vi "RC steering control.vi"(8 "filterd chan 0":dbl, 9 "Control with RC":bool, 10 "Duty Cycle in":dbl(slide) scale=0.0..1.0, 11 "Switch direction in":bool) -> (0 "Switch direction out":bool, 2 "Duty Cycle out":dbl)   [LabVIEW 2016]
doc: "Input\nChannel 0 data\nControl with RC\nDuty cycle\n\nOutput\nSwitch direction out\nDuty cycle out\n\nThis VI interpolates the value from the right joystick of the RC controller and produces a duty cycle between 0 and 0.2. The direction of the motor is determined by the Switch direction out boolean. If the RC switch on channel 6 is not in position 2, we send the duty cycle from the front panel."
uses:
  <vilib>/gmath/NI_Gmath.lvlib
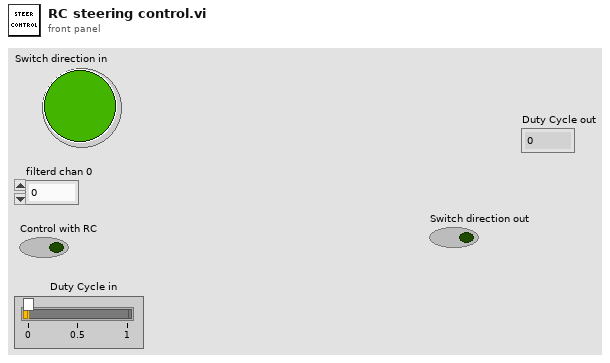
[diagram p1: front panel]
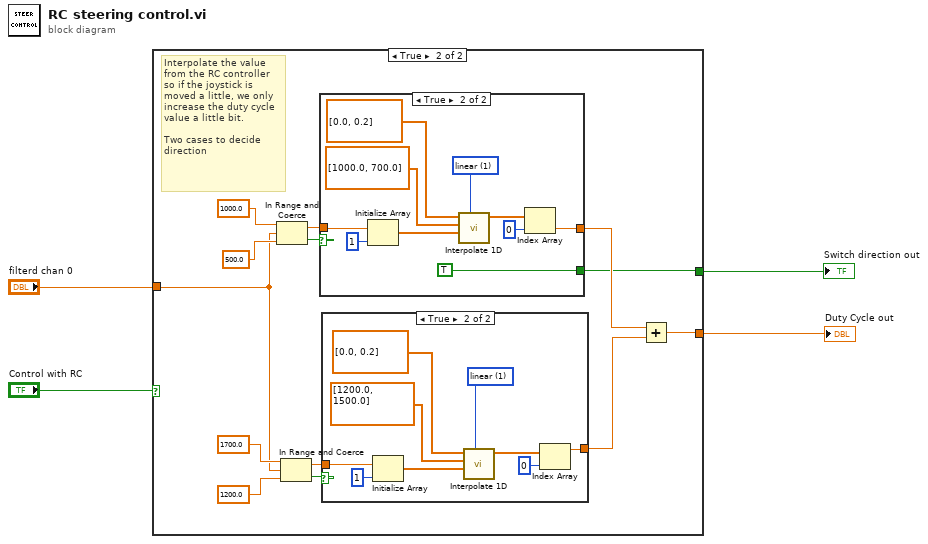
[diagram p0: block diagram]
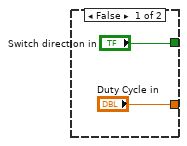
[diagram p2: hidden frame]
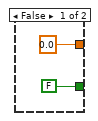
[diagram p3: hidden frame]
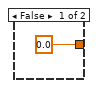
[diagram p4: hidden frame]
diagram:
  n1 = case shown="True" "Control with RC" {
    tunnel: ["Duty Cycle in" w9] -> w1
    tunnel: "filterd chan 0" -> [_ w8]
    tunnel: ["Switch direction in" w7] -> w4
    frame False {
    }
    frame True {
      # "Interpolate the value\nfrom the RC controller\nso if the joystick is\nmoved a little, we only\nincrease the duty cycle\nvalue a little bit. \n\nTwo cases to decide\ndirection"
      n2 = In Range and Coerce(upper limit=1000.0, x=w8, lower limit=500.0) -> (coerced(x)=w14:dbl, In Range?=w13:bool)
      n3 = In Range and Coerce(upper limit=1700.0 ("y"), x=w8, lower limit=1200.0 ("y")) -> (coerced(x)=w12:dbl, In Range?=w15:bool)
      n4 = case shown="True" w13 {
        tunnel: w14 -> [_ w28]
        tunnel: [0.0 w22] -> w11
        tunnel: [FALSE TRUE] -> w7
        frame False {
        }
        frame True {
          w25 = 1 items=["nearest", "linear", "spline", "cubic Hermite", "Lagrange"] ("method")
          n5 = Initialize Array(w28, 1 ("dimension size")) -> (w27:dbl[])
          n6 = call <vilib>:"Interpolate 1D.vi"("method"=w25, "xi"=w27, "X"=dbl[] [1000.0, 700.0], "Y"=dbl[] [0.0, 0.2]) -> ("yi"=w23:dbl[])  [unwired: 5 in, 2 out]
          n7 = Index Array(array=w23, index=0) -> (element=w22:dbl)
        }
      }
      n8 = case shown="True" w15 {
        tunnel: [0.0 w33] -> w10
        tunnel: w12 -> [_ w38]
        frame False {
        }
        frame True {
          w36 = 1 items=["nearest", "linear", "spline", "cubic Hermite", "Lagrange"] ("method")
          n9 = Initialize Array(w38, 1 ("dimension size")) -> (w40:dbl[])
          n10 = call <vilib>:"Interpolate 1D.vi"("method"=w36, "xi"=w40, "X"=dbl[] [1200.0, 1500.0], "Y"=dbl[] [0.0, 0.2]) -> ("yi"=w34:dbl[])  [unwired: 5 in, 2 out]
          n11 = Index Array(array=w34, index=0) -> (element=w33:dbl)
        }
      }
      n12 = Add(x=w11, y=w10) -> (x+y=w9:dbl)
    }
  }
  "Switch direction out" <- w4
  "Duty Cycle out" <- w1
